vi "Get Sender.vi"(11 "Teardown Error Msg in":refnum<class "Teardown Error Msg.lvclass">) -> (2 "Sender":refnum<class "Sender.lvclass">)   [LabVIEW 2020, in "jettl.lvlib" / "Teardown Error Msg.lvlib" / "Teardown Error Msg.lvclass"]
uses:
  Teardown Error Msg.lvclass
  Sender/Sender/Sender.lvclass
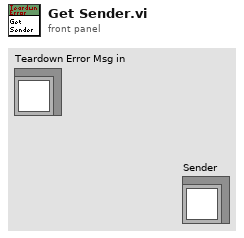
[diagram p1: front panel]
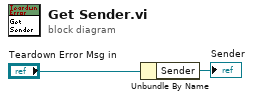
[diagram p0: block diagram]
diagram:
  n1 = Unbundle By Name("Teardown Error Msg in") -> ("Sender"=→"Sender":refnum<class "Sender.lvclass">)
